vi "Is POV Empty.vi"(11 "POVs":i16[](array[numeric])) -> (3 "Numeric":i16)   [LabVIEW 2019, in "Joysticks.lvlib" / "Two Drivers.lvclass"]
uses:
  Two Drivers.lvclass
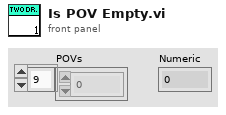
[diagram p1: front panel]
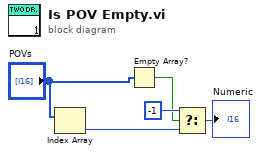
[diagram p0: block diagram]
diagram:
  n1 = Index Array(array="POVs") -> (element=w1:i16)  [unwired: 1 in]
  n2 = Empty Array?(array="POVs") -> (empty?=w4:bool)
  n3 = Select(t=i16 -1, s=w4, f=w1) -> (s? t:f=→"Numeric":i16)
